vi "S2C_FORNAX_Proc_Request.vi"(7 "Local?":bool, 8 "Error In":errorcluster, 9 "CmdString":string, 10 "Command":string, 11 "Timeout":dbl) -> (0 "Error Out":errorcluster, 3 "Response":string)   [LabVIEW 2015]
uses:
  S2C_FORNAX_Proc_Globals.vi
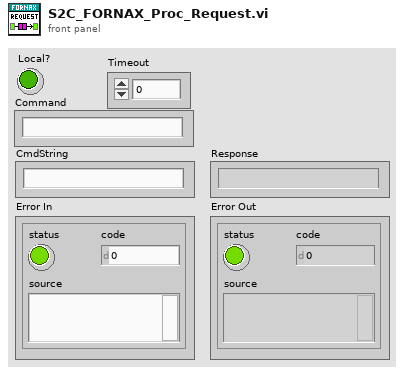
[diagram p1: front panel]
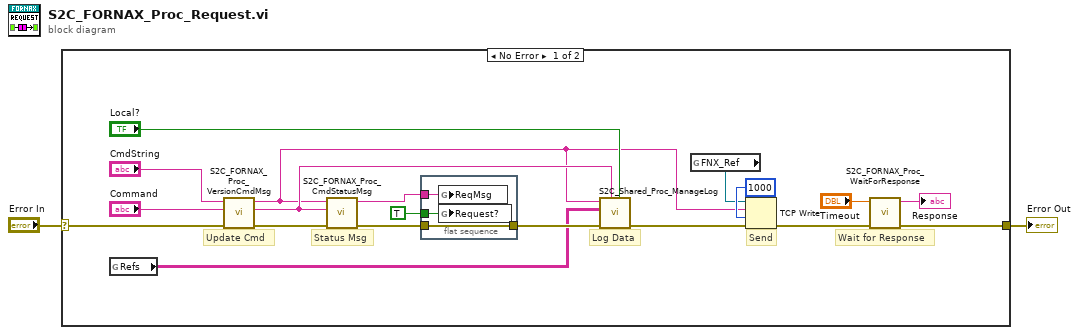
[diagram p0: block diagram]
diagram:
  n1 = case shown="No Error" "Error In" {
    selector: "Error In" -> [w8 w25]
    tunnel: [w10 w25] -> w1
    frame No Error {
      # "Update Cmd"
      # "Log Data"
      # "Wait for Response"
      # "Status Msg"
      # "Send"
      n2 = global read "S2C_FORNAX_Proc_Globals.vi" "Refs"() -> (w9:string[][])
      n3 = call "S2C_FORNAX_Proc_VersionCmdMsg.vi"("Error In"=w8, "Cmd In"="Command", "JSON In"="CmdString") -> ("Error Out"=w5:errorcluster, "Cmd Out"=w4:string, "JSON Out"=w3:string)  [unwired: 6 in]
      n4 = call "S2C_FORNAX_Proc_CmdStatusMsg.vi"("Error In"=w5, "CmdMsg"=w4, "CmdString"=w3) -> ("Error Out"=w20:errorcluster, "StatusMsg"=w19:string)  [unwired: 7 in]
      n5 = flat-sequence {
        tunnel: w20 -> [w24]
        tunnel: [w24] -> w14
        tunnel: w19 -> [w23]
        tunnel: TRUE ("Request?") -> [w22]
        frame #0 {
          n6 = global write "S2C_FORNAX_Proc_Globals.vi" "ReqMsg"(w23) -> ()
          n7 = global write "S2C_FORNAX_Proc_Globals.vi" "Request?"(w22) -> ()
        }
      }
      n8 = call "S2C_Shared_Proc_ManageLog.vi"("Local?"="Local?", "Command"=w4, "Error In"=w14, "Refs"=w9, "Data In"=w3) -> ("Error Out"=w13:errorcluster)  [unwired: 5 in, 1 out]
      n9 = global read "S2C_FORNAX_Proc_Globals.vi" "FNX_Ref"() -> (w15:refnum<k5>)
      n10 = TCP Write(connection ID=w15, data in=w3, error in (no error)=w13, 9:1000 ("timeout ms (25000)")) -> (error out=w17:errorcluster)  [unwired: 2 out]
      n11 = call "S2C_FORNAX_Proc_WaitForResponse.vi"("Error In"=w17, "Timeout"="Timeout") -> ("Error Out"=w10:errorcluster, "Response"=→"Response":string)  [unwired: 8 in]
    }
    frame Error {
    }
  }
  "Error Out" <- w1
